vi "ToString.vi"(8 "error in (no error)":errorcluster, 11 "U32 D Element in":refnum<class "Bool D Element.lvclass">) -> (0 "error out":errorcluster, 2 "String":string, 3 "U32 D Element out":refnum<class "Bool D Element.lvclass">)   [LabVIEW 2020, in "D Datagrid Library.lvlib" / "Bool D Element.lvclass"]
uses:
  Bool D Element.lvclass
  Bool D Element.lvclass/Bool D Element.ctl
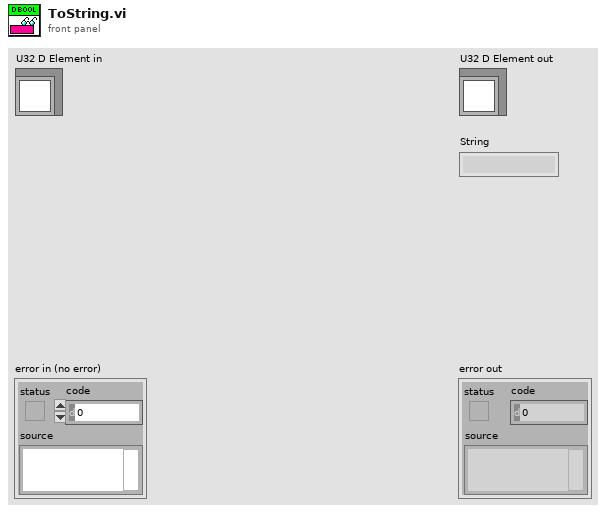
[diagram p1: front panel]
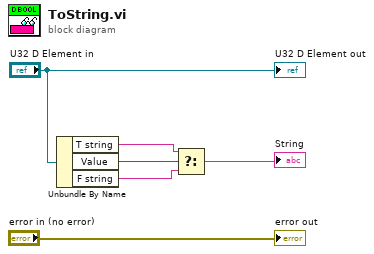
[diagram p0: block diagram]
diagram:
  n1 = Unbundle By Name("U32 D Element in") -> ("T string"=w2:string, "Value"=w4:bool, "F string"=w1:string)
  n2 = Select(t=w2, s=w4, f=w1) -> (s? t:f=→"String":string)
  "error out" <- "error in (no error)"
  "U32 D Element out" <- "U32 D Element in"
